vi "To Value.vi"(8 "error in (no error)":errorcluster, 10 "PV Data in":refnum<class "PV Data.lvclass">, 11 "NT Base in":refnum<class "NT Base.lvclass">) -> (0 "error out":errorcluster, 2 "PV Data out":refnum<class "PV Data.lvclass">, 3 "NT Base out":refnum<class "NT Base.lvclass">)   [LabVIEW 2020, in "PV Access.lvlib" / "PV Data.lvlib" / "NT Base.lvclass"]
uses:
  NT Base.lvclass
  PV Data/PV Data.lvclass
  bf4cc474-99ee-445c-a1f4-9c617dff90c8.vi
  92fae744-0f71-400a-bf7c-acbbe739e743.vi
  PV Data.lvlib
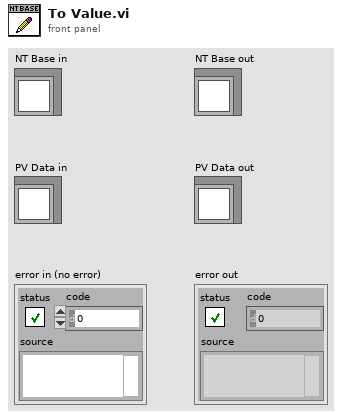
[diagram p1: front panel]
types:
  T1 = typedef "PV Access.lvlib/PV Data.lvlib/Type Code.ctl" = enum8{"Null", "Bool", "BoolA", "Int8", "Int8A", "Int16", "Int16A", "Int32", "Int32A", "Int64", "Int64A", "UInt8", "UInt8A", "UInt16", "UInt16A", "UInt32", "UInt32A", "UInt64", "UInt64A", "Float32", "Float32A", "Float64", "Float64A", "String", "StringA", "Struct", "StructA", "Union", "UnionA", "Any", "AnyA"}
  T2 = typedef "PV Access.lvlib/PV Data.lvlib/Alarm.ctl" = cluster{"Severity":T3, "Status":T4, "Message":string}
  T3 = typedef "PV Access.lvlib/PV Data.lvlib/Alarm Severity.ctl" = enum32{"no", "minor", "major", "record", "invalid", "undefined", ""}
  T4 = typedef "PV Access.lvlib/PV Data.lvlib/Alarm Status.ctl" = enum32{"no", "device", "driver", "record", "db", "conf", "undefined", "client"}
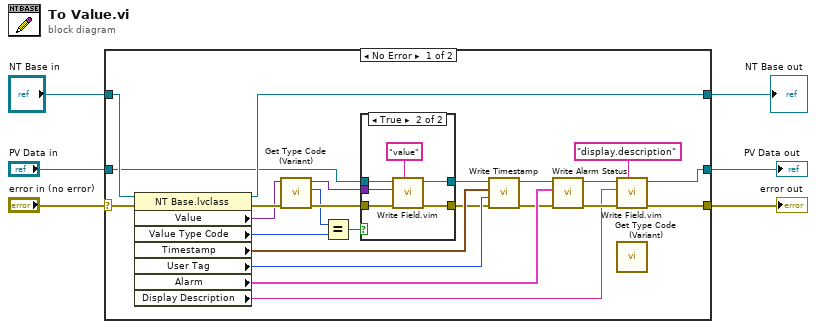
[diagram p0: block diagram]
diagram:
  n1 = case shown="No Error" "error in (no error)" {
    selector: "error in (no error)" -> [w29 w41]
    tunnel: [w16 w41] -> w5
    tunnel: [w27 w40] -> w3
    tunnel: "NT Base in" -> [w30 w40]
    tunnel: [w15 w39] -> w2
    tunnel: "PV Data in" -> [w24 w39]
    frame No Error {
      n2 = property class="NT Base.lvclass"(reference=w30, error in=w29) -> (reference out=w27:refnum<class "NT Base.lvclass">, error out=w12:errorcluster, "Value"=w11:variant, "Value Type Code"=w9:T1, "Timestamp"=w26:timestamp, "User Tag"=w28:i32, "Alarm"=w22:T2, "Display Description"=w17:string)
      n3 = call "Get Type Code (Variant).vi"("error in (no error)"=w12, "value"=w11) -> ("error out"=w13:errorcluster, "type code"=w8:T1, "value dup"=w10:variant)  [unwired: 5 in]
      n4 = Equal?(x=w8, y=w9) -> (x = y?=w7:bool)
      n5 = case shown="True" w7 {
        tunnel: [w31 w38] -> w25
        tunnel: w24 -> [w32 w37]
        tunnel: [w32 w36] -> w23
        tunnel: w13 -> [w31 w34]
        tunnel: w10 -> [_ w33]
        frame False {
        }
        frame True {
          n6 = call "Write Field.vim"("field name"="value", "error in"=w34, "value in"=w33, "PV Data in"=w37) -> ("error out"=w38:errorcluster, "PV Data out"=w36:refnum<class "PV Data.lvclass">)  [unwired: 5 in, 1 out]
        }
      }
      n7 = call "Write Timestamp.vi"("error in"=w25, "user tag"=w28, "timestamp"=w26, "PV Data in"=w23) -> ("error out"=w20:errorcluster, "PV Data out"=w21:refnum<class "PV Data.lvclass">)  [unwired: 6 in]
      n8 = call "Write Alarm Status.vi"("error in"=w20, "alarm status"=w22, "PV Data in"=w21) -> ("error out"=w18:errorcluster, "PV Data out"=w19:refnum<class "PV Data.lvclass">)  [unwired: 7 in]
      n9 = call "Write Field.vim"("field name"="display.description", "error in"=w18, "value in"=w17, "PV Data in"=w19) -> ("error out"=w16:errorcluster, "PV Data out"=w15:refnum<class "PV Data.lvclass">)  [unwired: 5 in, 1 out]
      n10 = call "Get Type Code (Variant).vi"() -> ()  [unwired: 7 in, 3 out]
    }
    frame Error {
    }
  }
  "error out" <- w5
  "NT Base out" <- w3
  "PV Data out" <- w2
